vi "get reignition voltage.vi"(5 "stable rf gen voltage":dbl, 7 "polarimeter threshold":dbl, 9 "reignitor task":refnum<k21>, 10 "polarimeter task":refnum<k21>, 11 "rf generator task":refnum<k21>) -> (0 "Min Reignition Voltage":dbl, 1 "reignitor task":refnum<k21>, 2 "polarimeter task":refnum<k21>, 3 "rf generator task":refnum<k21>)   [LabVIEW 2018]
uses:
  <vilib>/DAQmx/write.llb/DAQmx Write (Analog DBL 1Chan 1Samp).vi
  a8074ea1-1c0a-4296-9646-7d5559e3d868.vi
  b15d0405-1705-47a4-a36f-a0cd54eda9bd.vi
  37882e86-5f32-4f0b-bb7e-73c8138da298.vi
  <vilib>/DAQmx/read.llb/DAQmx Read (Analog DBL 1Chan 1Samp).vi
  <vilib>/DAQmx/miscellaneous.llb/DAQmx Fill In Error Info.vi
panel:
  out "Waveform Chart":dbl(graph)
  out "current rf voltage in":dbl
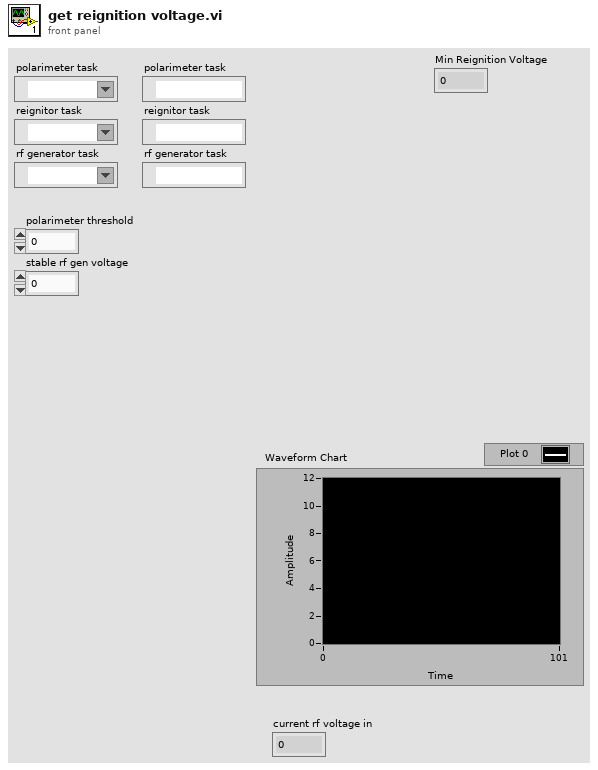
[diagram p1: front panel]
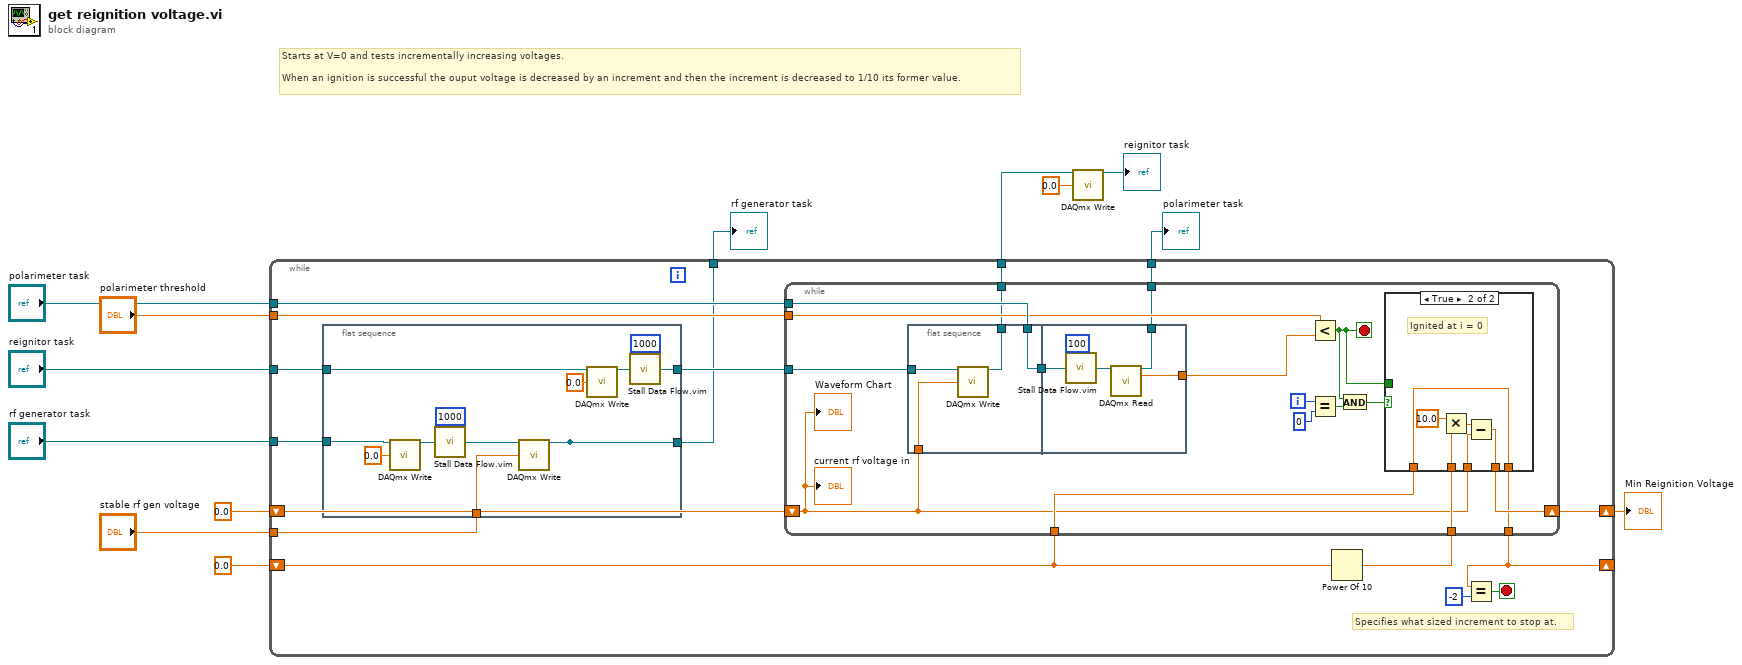
[diagram p0: block diagram]
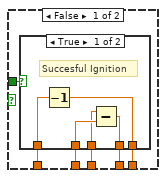
[diagram p2: hidden frame]
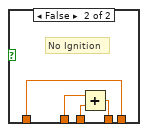
[diagram p3: hidden frame]
diagram:
  # "Starts at V=0 and tests incrementally increasing voltages.\n\nWhen an ignition is successful the ouput voltage is decreased by an increment and then the increment is decreased to 1/10 its former value."
  n1 = while {
    tunnel: "polarimeter task" -> [w22]
    shift-right: [w26] -> w13
    shift-left: 0.0 -> [w19]
    tunnel: "reignitor task" -> [w29]
    shift-right: [w23] -> _
    shift-left: 0.0 -> [w25]
    tunnel: "polarimeter threshold" -> [w20]
    tunnel: "rf generator task" -> [w18]
    tunnel: "stable rf gen voltage" -> [w17]
    tunnel: [w16] -> w3
    tunnel: [w15] -> w5
    tunnel: [w14] -> w4
    stop <- w27 stop-if-true
    # "Specifies what sized increment to stop at."
    n2 = flat-sequence {
      tunnel: w29 -> [w39]
      tunnel: [w38] -> w21
      tunnel: w18 -> [w33]
      tunnel: w17 -> [w32]
      tunnel: [w31] -> _
      tunnel: [w31] -> w14
      frame #0 {
        n3 = call-poly <vilib>:"DAQmx Write.vi"("task/channels in"=w33, "data"=0.0) -> ("task out"=w36:refnum<k21>)  [unwired: 11 in, 2 out]
        n4 = call "Stall Data Flow.vim"("value in"=w36, "milliseconds to wait"=u32 1000) -> ("value out"=w37:refnum<k21>)  [unwired: 1 out]
        n5 = call-poly <vilib>:"DAQmx Write.vi"("task/channels in"=w37, "data"=w32) -> ("task out"=w31:refnum<k21>)  [unwired: 11 in, 2 out]
        n6 = call-poly <vilib>:"DAQmx Write.vi"("task/channels in"=w39, "data"=0.0) -> ("task out"=w41:refnum<k21>)  [unwired: 11 in, 2 out]
        n7 = call "Stall Data Flow.vim"("value in"=w41, "milliseconds to wait"=u32 1000) -> ("value out"=w38:refnum<k21>)  [unwired: 1 out]
      }
    }
    n8 = Power Of 10(x=w25) -> (10^x=w24:dbl)
    n9 = while {
      tunnel: w22 -> [w50]
      tunnel: w21 -> [w51]
      shift-right: [w53] -> w26
      shift-left: w19 -> [w45]
      tunnel: w24 -> [w54]
      tunnel: w25 -> [w48]
      tunnel: [w52] -> w23
      tunnel: w20 -> [w44]
      tunnel: [w43] -> w16
      tunnel: [w42] -> w15
      i -> [w58]
      stop <- w46 stop-if-true
      n10 = flat-sequence {
        tunnel: w45 -> [w62]
        tunnel: w51 -> [w61]
        tunnel: w50 -> [w60]
        tunnel: [w60] -> w49
        tunnel: [w59] -> w43
        tunnel: w49 -> [w66]
        tunnel: [w65] -> w47
        tunnel: [w63] -> w42
        frame #0 {
          n11 = call-poly <vilib>:"DAQmx Write.vi"("task/channels in"=w61, "data"=w62) -> ("task out"=w59:refnum<k21>)  [unwired: 11 in, 2 out]
        }
        frame #1 {
          n12 = call "Stall Data Flow.vim"("value in"=w66, "milliseconds to wait"=u32 100) -> ("value out"=w67:refnum<k21>)  [unwired: 1 out]
          n13 = call-poly <vilib>:"DAQmx Read.vi"("task/channels in"=w67) -> ("task out"=w63:refnum<k21>, "data"=w65:dbl)  [unwired: 12 in, 1 out]
        }
      }
      n14 = Less?(x=w44, y=w47) -> (x < y?=w46:bool)
      n15 = Equal?(x=w58, y=0) -> (x = y?=w56:bool)
      n16 = And(x=w46, y=w56) -> (x .and. y?=w55:bool)
      n17 = case shown="True" w55 {
        tunnel: w54 -> [w71 w88]
        tunnel: w45 -> [w72 w85]
        tunnel: [w73 w84] -> w53
        tunnel: w48 -> [w70 w83]
        tunnel: [w69 w83] -> w52
        tunnel: w46 -> [w68 _]
        frame False {
          n18 = case shown="True" w68 {
            tunnel: [w78 w81] -> w73
            tunnel: w72 -> [w74 w80]
            tunnel: w71 -> [w75 w79]
            tunnel: w70 -> [w77 w82]
            tunnel: [w76 w82] -> w69
            frame True {
              # "Succesful Ignition"
              n19 = Decrement(x=w77) -> (x-1=w76:dbl)
              n20 = Subtract(x=w74, y=w75) -> (x-y=w78:dbl)
            }
            frame False {
              # "No Ignition"
              n21 = Add(x=w79, y=w80) -> (x+y=w81:dbl)
            }
          }
        }
        frame True {
          # "Ignited at i = 0"
          n22 = Multiply(x=10.0, y=w88) -> (x*y=w86:dbl)
          n23 = Subtract(x=w86, y=w85) -> (x-y=w84:dbl)
        }
      }
      "Waveform Chart" <- w45
      "current rf voltage in" <- w45
    }
    n24 = Equal?(x=w23, y=-2) -> (x = y?=w27:bool)
  }
  "Min Reignition Voltage" <- w13
  "polarimeter task" <- w5
  "rf generator task" <- w4
  n25 = call-poly <vilib>:"DAQmx Write.vi"("task/channels in"=w3, "data"=0.0) -> ("task out"=→"reignitor task":refnum<k21>)  [unwired: 11 in, 2 out]
